vi "LJM logger configuration panel.vi"(0 "Working Directory":path, 1 "Current Device Connection In":T1={"Device Type"="ANY", "Connection Type"="ANY", "Serial Number"=0}, 5 "App name":string="LJM_New_Open", 7 "Handle In":i32, 9 "Program Configs":T2={"Data File Prefix"="", "Scan Rate (Hz)"=0.0, "Graph History"=0, "# Channels"=0, "Disable Scaling"=FALSE, "Max File Size (Bytes)"=0, "Channel Setup"={"Name"=["AIN0", "AIN1", "AIN2", "AIN3", "AIN4", "AIN5", "AIN6", "AIN7", "AIN8", "AIN9", "AIN10", "AIN11", "AIN12", "AIN13", "AIN14", "AIN15"], "", "Scaling Equation"=["y=a", "y=b", "y=c", "y=d", "y=e", "y=f", "y=g", "y=h", "y=i", "y=j", "y=k", "y=l", "y=m", "y=n", "y=o", "y=p"], "", "Graph?"=[TRUE, TRUE, TRUE, TRUE, FALSE, FALSE, FALSE, FALSE, FALSE, FALSE, FALSE, FALSE, FALSE, FALSE, FALSE, FALSE]}, "Interval (ms)"=0, "Write To File"=FALSE, "Log Every n Scans"=0}, 11 "Device Open Params In":T4, 13 "Streaming App?":bool=TRUE) -> (4 "Working Directory Out":path caption="Current Working Directory", 8 "Handle Out":i32, 10 "Program Configs Out":T2={"Data File Prefix"="", "Scan Rate (Hz)"=0.0, "Graph History"=0, "# Channels"=0, "Disable Scaling"=FALSE, "Max File Size (Bytes)"=0, "Channel Setup"={"Name"=["AIN0", "AIN1", "AIN2", "AIN3", "AIN4", "AIN5", "AIN6", "AIN7", "AIN8", "AIN9", "AIN10", "AIN11", "AIN12", "AIN13", "AIN14", "AIN15"], "", "Scaling Equation"=["y=a", "y=b", "y=c", "y=d", "y=e", "y=f", "y=g", "y=h", "y=i", "y=j", "y=k", "y=l", "y=m", "y=n", "y=o", "y=p"], "", "Graph?"=[TRUE, TRUE, TRUE, TRUE, FALSE, FALSE, FALSE, FALSE, FALSE, FALSE, FALSE, FALSE, FALSE, FALSE, FALSE, FALSE]}, "Interval (ms)"=0, "Write To File"=FALSE, "Log Every n Scans"=0}, 12 "Current Device Connection Out":T1={"Device Type"="ANY", "Connection Type"="ANY", "Serial Number"=0} caption="Current Device Connection", 15 "Device Open Params Out":T4)   [LabVIEW 2026]
uses:
  Common Logger Controls/Device Open Config Cluster.ctl
  Common Logger Controls/Currently Opened Device Params.ctl
  Common Logger Controls/Program Config Cluster.ctl
  Common Logger Controls/Channel Setup.ctl
  <vilib>/Platform/browser.llb/Open URL in Default Browser (string).vi
panel:
  in  "Identifier":string(combo)="ANY"
  in  "Change Working Directory":bool
  in  "Load Factory I/O Configuration":bool
  in  "Write?":bool[](array[boolean])=[FALSE, FALSE, FALSE, FALSE, FALSE, FALSE, FALSE, FALSE, FALSE, FALSE, FALSE, FALSE]
  in  "Values":dbl[](array[numeric])=[0.0, 0.0, 0.0, 0.0, 0.0, 0.0, 0.0, 0.0, 0.0, 0.0, 0.0, 0.0] format="%.2f"
  in  "Registers":string[](array[string])=["DAC0", "DAC1", "AIN_ALL_RESOLUTION_INDEX", "AIN_ALL_RANGE", "AIN_ALL_NEGATIVE_CH", "AIN0_RESOLUTION_INDEX", "AIN0_RANGE", "AIN0_NEGATIVE_CH", "AIN0_EF_INDEX", "AIN0_EF_CONFIG_A", "DIO4_EF_INDEX", "DIO4_EF_ENABLE"]
  in  "Save Power-Up I/O Configuration":bool
  in  "Open Modbus Map":bool
  in  "Write Device Registers":bool
  in  "Redo Device Open":bool
  in  "Connection Type Config":string(combo)="ANY" caption="Connection Type"
  in  "Device Type Config":string(combo)="ANY" caption="Device Type"
  in  "Load New Program Configuration":bool
  in  "Save Program Configuration":bool
  out "Messages":string="No Error"
  in  "Exit":bool
  # "Device Open"
  # "Device I/O Configuration"
  # "Open a New Device Connection"
  # "Click \"?\" to open a link to the Modbus Map for detailed register information."
  # "Save the values of your front panel controls to file."
  # "Set the current device I/O configs as the power-up default"
  # "Load values for your front panel controls from file."
  # "Load and apply factory default I/O configs for the device."
  # "Program Working Directory"
  # "Change the directory where config files and log files are saved."
  # "Configuration Panel Messages"
  # "Open a new device connection using the parameters to the left"
  # "Program Configurations"
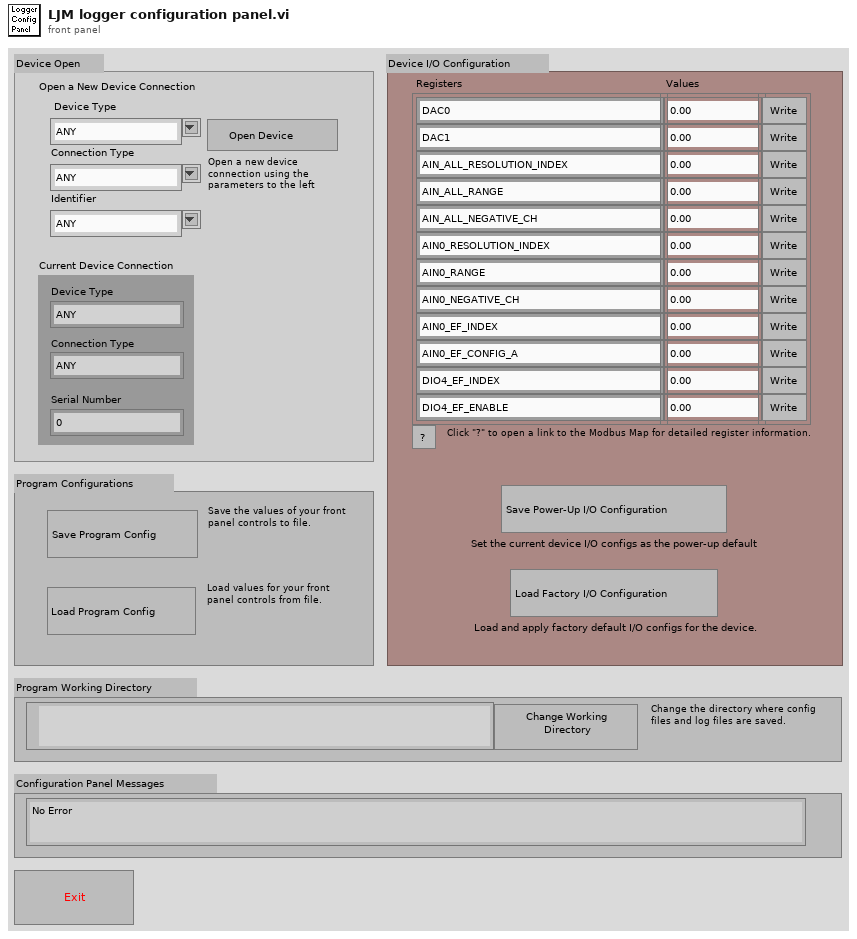
[diagram p1: front panel]
types:
  T1 = typedef "Currently Opened Device Params.ctl" = cluster{"Device Type":string, "Connection Type":string, "Serial Number":i32}
  T2 = typedef "Program Config Cluster.ctl" = cluster{"Data File Prefix":string, "Scan Rate (Hz)":dbl, "Graph History":i32, "# Channels":i32, "Disable Scaling":bool, "Max File Size (Bytes)":i32, "Channel Setup":T3, "Interval (ms)":u32, "Write To File":bool, "Log Every n Scans":i32}
  T3 = typedef "Channel Setup.ctl" = cluster{"Name":string[], string, "Scaling Equation":string[], string, "Graph?":bool[]}
  T4 = typedef "Device Open Config Cluster.ctl" = cluster{"Open Config Device Type":string, "Open Config Connection Type":string, "Open Config Identifier":string}
  T5 = cluster{"Data File Prefix":string, "Scan Rate (Hz)":dbl, "Graph History":i32, "# Channels":i32, "Disable Scaling":bool, "Max File Size (Bytes)":i32, "Channel Setup 2":T3, "Interval (ms)":u32, "Write To File":bool, "Log Every n Scans":i32}
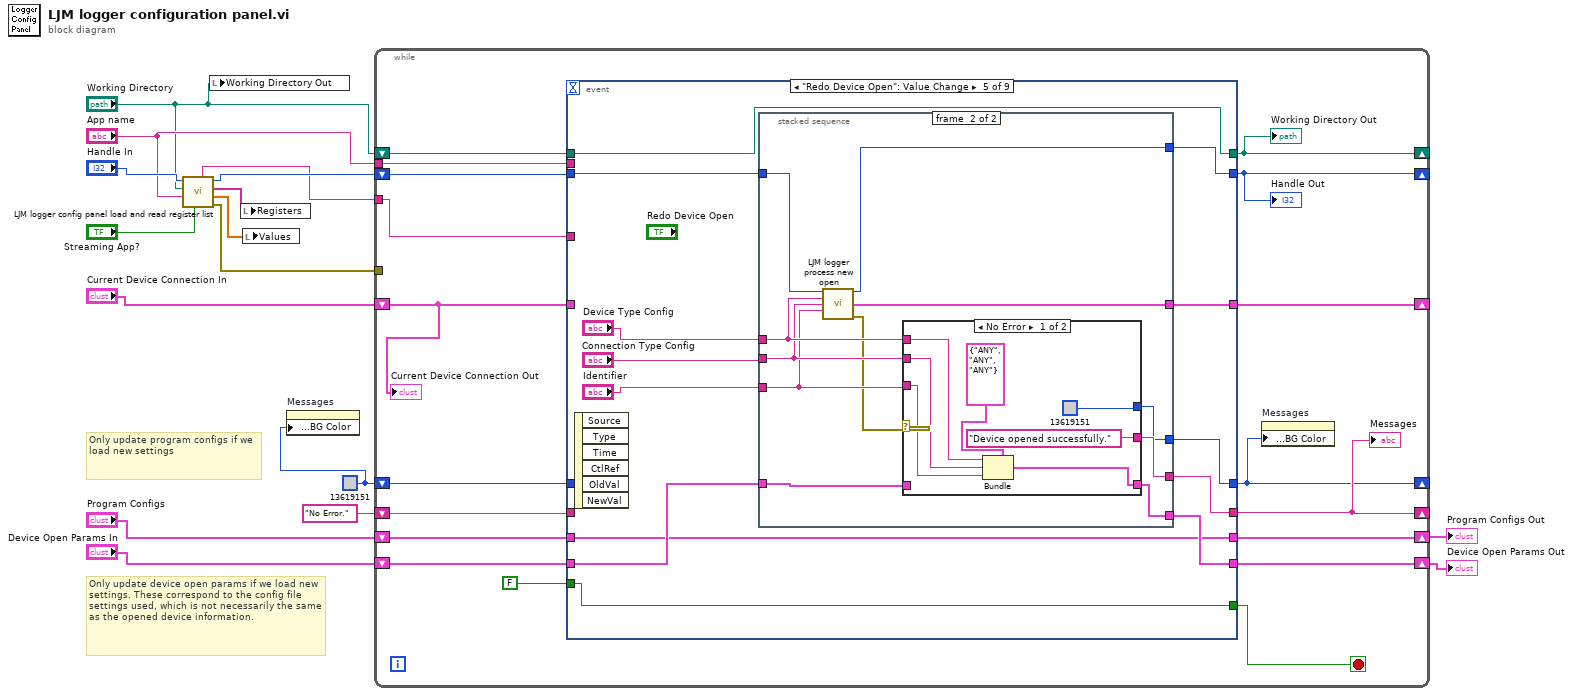
[diagram p0: block diagram]
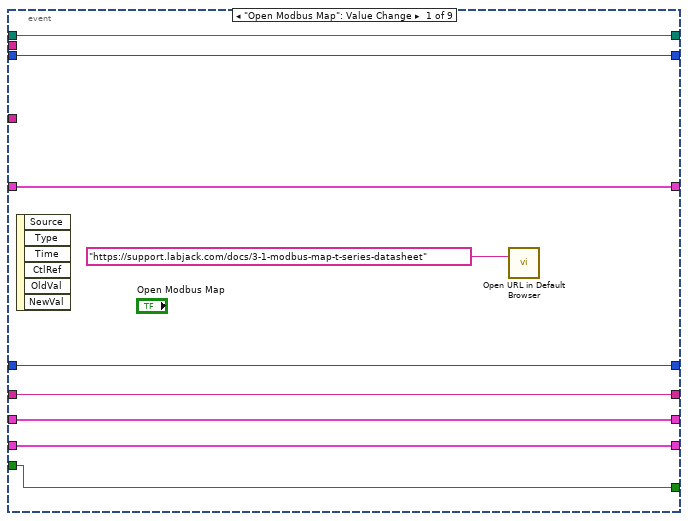
[diagram p2: hidden frame]
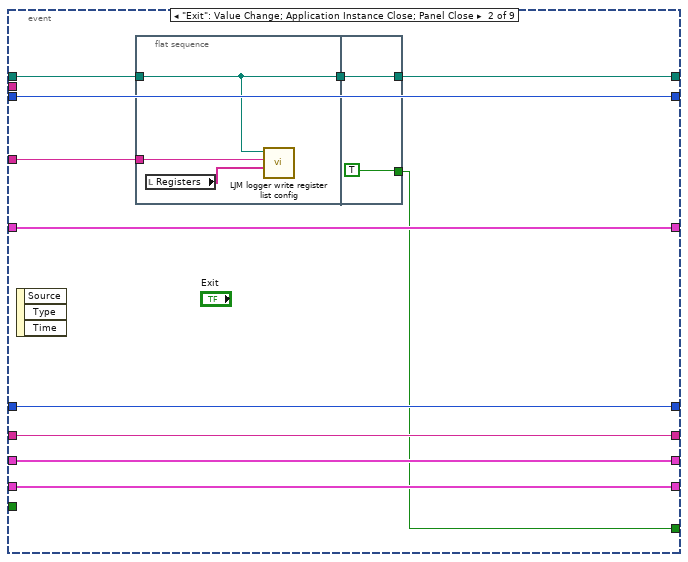
[diagram p3: hidden frame]
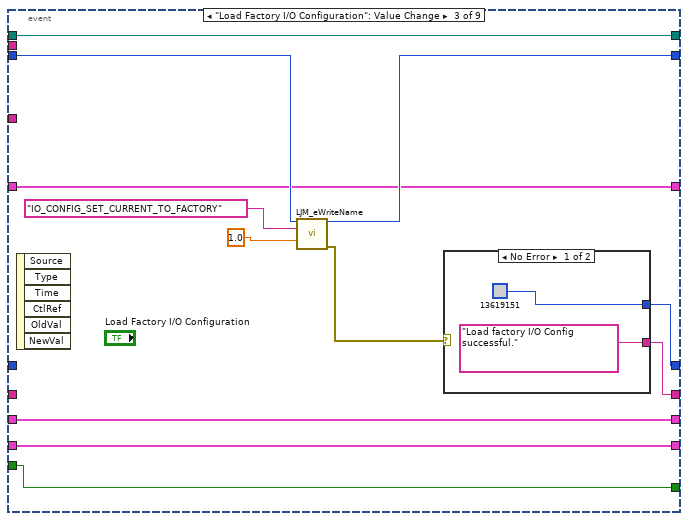
[diagram p4: hidden frame]
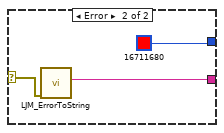
[diagram p5: hidden frame]
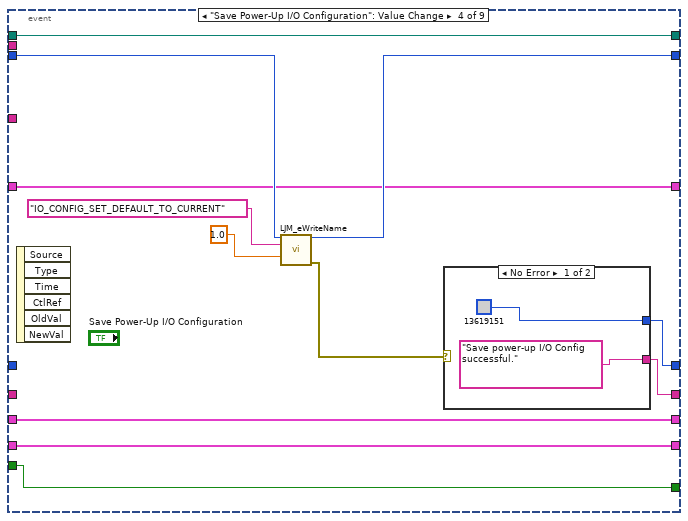
[diagram p6: hidden frame]
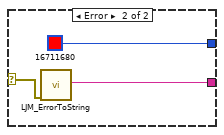
[diagram p7: hidden frame]
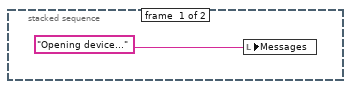
[diagram p8: hidden frame]
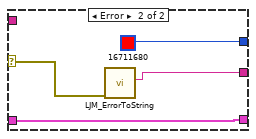
[diagram p9: hidden frame]
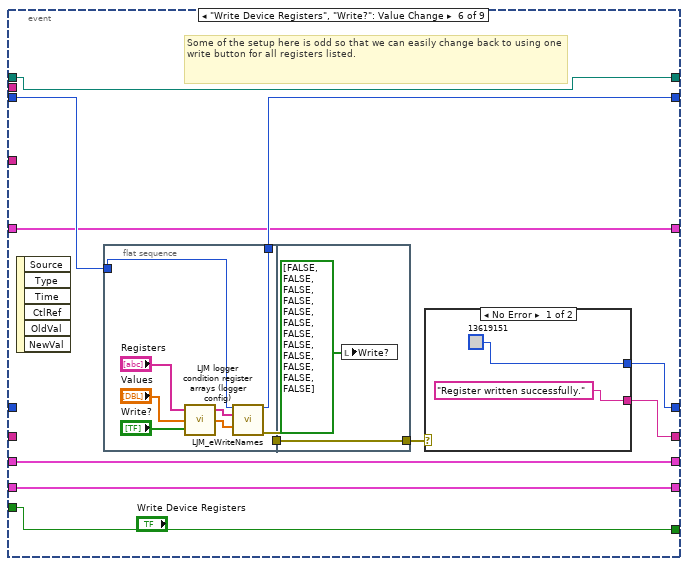
[diagram p10: hidden frame]
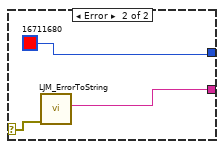
[diagram p11: hidden frame]
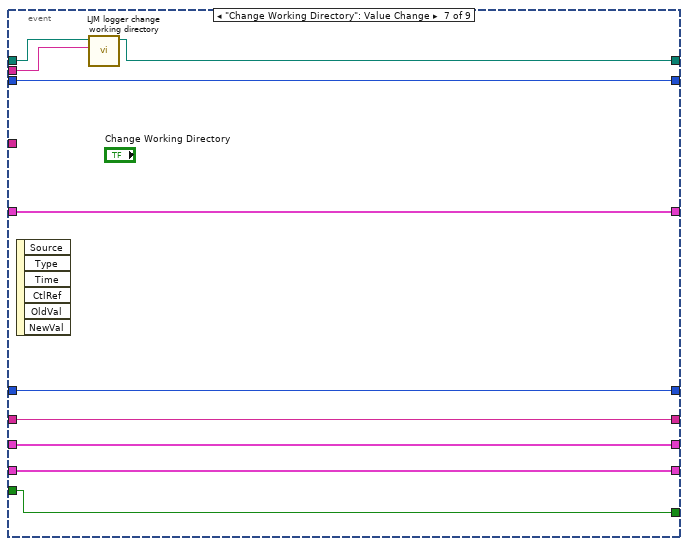
[diagram p12: hidden frame]
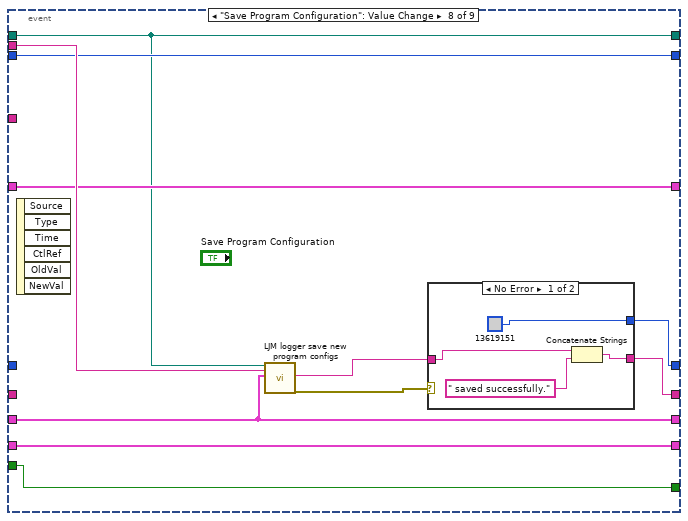
[diagram p13: hidden frame]
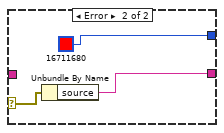
[diagram p14: hidden frame]
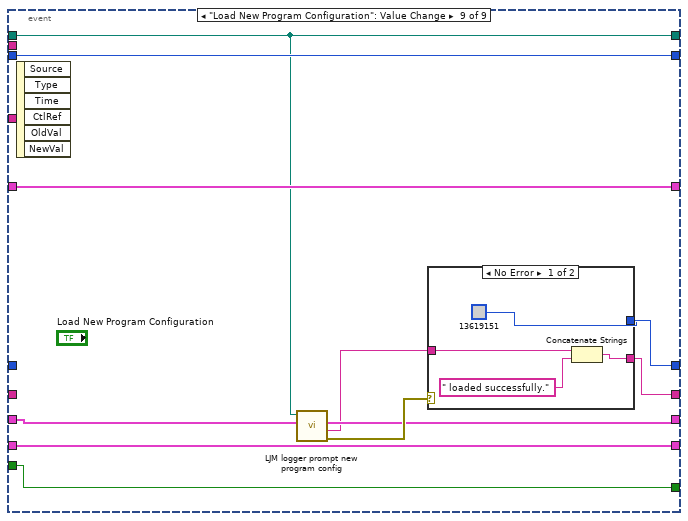
[diagram p15: hidden frame]
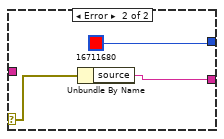
[diagram p16: hidden frame]
diagram:
  w2 = u32 13619151
  # "Only update program configs if we load new settings"
  # "Only update device open params if we load new settings. These correspond to the config file settings used, which is not necessarily the same as the opened device information."
  n1 = call "LJM logger config panel load and read register list.vi"("Streaming App?"="Streaming App?", "App name"="App name", "Working Directory"="Working Directory", "Handle In"="Handle In") -> ("Error Out"=w6:errorcluster, "Register Values"=w7:dbl[], "Register List"=w8:string[], "Handle Out"=w9:i32, "Register List Config Filename"=w4:string)  [unwired: 3 in]
  n2 = local write "Working Directory Out"("Working Directory") -> ()
  n3 = local write "Registers"(w8) -> ()
  n4 = local write "Values"(w7) -> ()
  n5 = property on="Messages" class="Str"("Text.Text Colors:BG Color"=w2) -> ()  [unwired: 2 in, 2 out]
  n6 = while {
    tunnel: "App name" -> [w32]
    shift-right: [w29] -> w14
    shift-left: "Device Open Params In" -> [w34]
    shift-right: [w21] -> w12
    shift-left: "Program Configs" -> [w30]
    shift-right: [w27] -> _
    shift-left: w9 -> [w33]
    shift-right: [w24] -> _
    shift-left: "No Error." ("source") -> [w25]
    shift-right: [w23] -> _
    shift-left: w2 -> [w26]
    shift-right: [w20] -> _
    shift-left: "Current Device Connection In" -> [w17]
    tunnel: w6 -> [_]
    tunnel: w4 -> [w19]
    shift-right: [w18] -> _
    shift-left: "Working Directory" -> [w31]
    stop <- w28 stop-if-true
    n7 = event shown="[4] \"Redo Device Open\": Value Change" {
      selector: _ -> [_ _ _ _ _ _ _ _ _]
      dyn-events: _ -> [_ _ _ _ _ _ _ _ _]
      timeout: _ -> [_ _ _ _ _ _ _ _ _]
      tunnel: w33 -> [w43 w53 w69 w82 w106 w139 w164 w169 w189]
      tunnel: [w43 w53 w68 w86 w101 w138 w164 w169 w189] -> w27
      tunnel: [w41 w51 w66 w84 w103 w136 w160 w175 w192] -> w24
      tunnel: [w42 w52 w65 w85 w102 w137 w161 w174 w191] -> w23
      tunnel: w34 -> [w40 w54 w64 w81 w105 w135 w158 w171 w190]
      tunnel: [w40 w54 w64 w81 w104 w135 w158 w171 w190] -> w29
      tunnel: w31 -> [w35 w48 w60 w77 w95 w130 w163 w166 w184]
      tunnel: w32 -> [_ _ _ _ _ _ w165 w172 _]
      tunnel: w30 -> [w38 w49 w62 w79 w96 w133 w159 w168 w193]
      tunnel: [w39 w46 w63 w80 w100 w134 w157 w170 w188] -> w28
      tunnel: w26 -> [w42 w52 _ _ _ _ w161 _ _]
      tunnel: w25 -> [w41 w51 _ _ _ _ w160 _ _]
      tunnel: FALSE ("Exit") -> [w39 _ w63 w80 w100 w134 w157 w170 w188]
      tunnel: [w37 w50 w61 w78 w97 w132 w156 w167 w186] -> w20
      tunnel: w17 -> [w37 w50 w61 w78 _ w132 w156 w167 w186]
      tunnel: [w38 w49 w62 w79 w96 w133 w159 w168 w187] -> w21
      tunnel: w19 -> [_ w47 _ _ _ _ _ _ _]
      tunnel: [w35 w45 w60 w77 w95 w130 w162 w166 w184] -> w18
      event "Open Modbus Map": Value Change {
        n8 = event-data() -> ()  [unwired: 1 in, 6 out]
        n9 = call-poly <vilib>:"Open URL in Default Browser.vi"("URL"="https://support.labjack.com/docs/3-1-modbus-map-t-series-datasheet") -> ()  [unwired: 5 in, 2 out]
      }
      event "Exit": Value Change; Application Instance Close; Panel Close {
        n10 = event-data() -> ()  [unwired: 1 in, 3 out]
        n11 = flat-sequence {
          tunnel: w48 -> [w55]
          tunnel: w47 -> [w57]
          tunnel: [w55] -> w44
          tunnel: [TRUE ("Exit")] -> w46
          tunnel: [w58] -> w45
          tunnel: w44 -> [w58]
          frame #0 {
            n12 = local read "Registers"() -> (w56:string[])
            n13 = call "LJM logger write register list config.vi"("Register List"=w56, "Filename"=w57, "Working Directory"=w55) -> ()  [unwired: 8 in, 1 out]
          }
          frame #1 {
          }
        }
      }
      event "Load Factory I/O Configuration": Value Change {
        n14 = event-data() -> ()  [unwired: 1 in, 6 out]
        n15 = call "LJM_eWriteName.vi"("Handle In"=w69, "Name"="IO_CONFIG_SET_CURRENT_TO_FACTORY", "Value"=1.0) -> ("Handle Out"=w68:i32, "error out"=w67:errorcluster)  [unwired: 11 in]
        n16 = case shown="No Error" w67 {
          selector: w67 -> [_ w76]
          tunnel: ["Load factory I/O Config successful." ("Messages") w75] -> w66
          tunnel: [u32 13619151 u32 16711680] -> w65
          frame No Error {
          }
          frame Error {
            n17 = call "LJM_ErrorToString.vi"("error in"=w76) -> ("String"=w75:string)  [unwired: 10 in]
          }
        }
      }
      event "Save Power-Up I/O Configuration": Value Change {
        n18 = event-data() -> ()  [unwired: 1 in, 6 out]
        n19 = call "LJM_eWriteName.vi"("Handle In"=w82, "Name"="IO_CONFIG_SET_DEFAULT_TO_CURRENT", "Value"=1.0) -> ("Handle Out"=w86:i32, "error out"=w83:errorcluster)  [unwired: 11 in]
        n20 = case shown="No Error" w83 {
          selector: w83 -> [_ w93]
          tunnel: [u32 13619151 u32 16711680] -> w85
          tunnel: ["Save power-up I/O Config  successful." ("Messages") w91] -> w84
          frame No Error {
          }
          frame Error {
            n21 = call "LJM_ErrorToString.vi"("error in"=w93) -> ("String"=w91:string)  [unwired: 10 in]
          }
        }
      }
      event "Redo Device Open": Value Change {
        n22 = event-data() -> ()  [unwired: 1 in, 6 out]
        n23 = stacked-sequence {
          tunnel: [_ w112] -> w101
          tunnel: "Device Type Config" -> [_ w116]
          tunnel: "Connection Type Config" -> [_ w115]
          tunnel: "Identifier" -> [_ w114]
          tunnel: w106 -> [_ w113]
          tunnel: [_ w118] -> w104
          tunnel: w105 -> [_ w117]
          tunnel: [_ w110] -> w103
          tunnel: [_ w109] -> w102
          tunnel: [_ w108] -> w97
          frame #0 {
            n24 = local write "Messages"("Opening device..." ("Messages")) -> ()
          }
          frame #1 {
            n25 = call "LJM logger process new open.vi"("Handle"=w113, "Device Type String"=w116, "Connection Type String"=w115, "Identifier String"=w114) -> ("Handle Out"=w112:i32, "Opened Device Params"=w108:T1, "error out"=w111:errorcluster)  [unwired: 9 in]
            n26 = case shown="No Error" w111 {
              selector: w111 -> [_ w128]
              tunnel: [w122 w129] -> w118
              tunnel: w116 -> [w125 _]
              tunnel: w115 -> [w124 _]
              tunnel: w114 -> [w123 _]
              tunnel: w117 -> [_ w129]
              tunnel: ["Device opened successfully." ("String") w127] -> w110
              tunnel: [u32 13619151 u32 16711680] -> w109
              frame No Error {
                n27 = Bundle(cluster=T4 {"Open Config Device Type"="ANY", "Open Config Connection Type"="ANY", "Open Config Identifier"="ANY"} ("Device Open Params In1"), "Open Config Device Type"=w125, "Open Config Connection Type"=w124, "Open Config Identifier"=w123) -> (w122:T4)
              }
              frame Error {
                n28 = call "LJM_ErrorToString.vi"("error in"=w128) -> ("String"=w127:string)  [unwired: 10 in]
              }
            }
          }
        }
      }
      event "Write Device Registers", "Write?": Value Change {
        # "Some of the setup here is odd so that we can easily change back to using one write button for all registers listed."
        n29 = event-data() -> ()  [unwired: 1 in, 6 out]
        n30 = flat-sequence {
          tunnel: w139 -> [w145]
          tunnel: [w144] -> w138
          tunnel: [w147] -> w131
          tunnel: [w150] -> w140
          tunnel: w131 -> [w150]
          frame #0 {
            n31 = call "LJM logger condition register arrays (logger config).vi"("Access?"="Write?", "Values"="Values", "Names"="Registers") -> ("Values Out"=w148:dbl[], "Names Out"=w146:string[])  [unwired: 1 in]
            n32 = call "LJM_eWriteNames.vi"("Handle In"=w145, "aNames"=w146, "aValuesIn"=w148) -> ("Handle Out"=w144:i32, "error out"=w147:errorcluster)  [unwired: 10 in, 1 out]
          }
          frame #1 {
            n33 = local write "Write?"(bool[] [FALSE, FALSE, FALSE, FALSE, FALSE, FALSE, FALSE, FALSE, FALSE, FALSE, FALSE, FALSE] ("Write?")) -> ()
          }
        }
        n34 = case shown="No Error" w140 {
          selector: w140 -> [_ w155]
          tunnel: [u32 13619151 u32 16711680] -> w137
          tunnel: ["Register written successfully." ("String") w154] -> w136
          frame No Error {
          }
          frame Error {
            n35 = call "LJM_ErrorToString.vi"("error in"=w155) -> ("String"=w154:string)  [unwired: 10 in]
          }
        }
      }
      event "Change Working Directory": Value Change {
        n36 = event-data() -> ()  [unwired: 1 in, 6 out]
        n37 = call "LJM logger change working directory.vi"("Application Name"=w165, "Working Directory In"=w163) -> ("Working Directory Out"=w162:path)  [unwired: 9 in]
      }
      event "Save Program Configuration": Value Change {
        n38 = event-data() -> ()  [unwired: 1 in, 6 out]
        n39 = call "LJM logger save new program configs.vi"("Working Directory"=w166, "App name"=w172, "Program Configs"=w168) -> ("Program Config Name"=w176:string, "error out"=w173:errorcluster)  [unwired: 14 in, 1 out]
        n40 = case shown="No Error" w173 {
          selector: w173 -> [_ w183]
          tunnel: w176 -> [w179 _]
          tunnel: [w178 w182] -> w175
          tunnel: [u32 13619151 u32 16711680] -> w174
          frame No Error {
            n41 = Concatenate Strings(w179, " saved successfully." ("String")) -> (w178:string)
          }
          frame Error {
            n42 = Unbundle By Name(w183) -> ("source"=w182:string)
          }
        }
      }
      event "Load New Program Configuration": Value Change {
        n43 = event-data() -> ()  [unwired: 1 in, 6 out]
        n44 = call "LJM logger prompt new program config.vi"("Program Configs In"=w193, "Working Directory In"=w184) -> ("error out"=w194:errorcluster, "New Program Config Name"=w185:string, "Program Configs Out"=w187:T5)  [unwired: 7 in]
        n45 = case shown="No Error" w194 {
          selector: w194 -> [_ w201]
          tunnel: w185 -> [w197 _]
          tunnel: [w196 w199] -> w192
          tunnel: [u32 13619151 u32 16711680] -> w191
          frame No Error {
            n46 = Concatenate Strings(w197, " loaded successfully." ("String")) -> (w196:string)
          }
          frame Error {
            n47 = Unbundle By Name(w201) -> ("source"=w199:string)
          }
        }
      }
    }
    "Messages" <- w24
    "Handle Out" <- w27
    "Working Directory Out" <- w18
    n48 = property on="Messages" class="Str"("Text.Text Colors:BG Color"=w23) -> ()  [unwired: 2 in, 2 out]
    "Current Device Connection Out" <- w17
  }
  "Device Open Params Out" <- w14
  "Program Configs Out" <- w12
